vi "Read Menu Name.vi"(8 "error in":errorcluster, 11 "Standard Engine Editor Node in":refnum<class "Standard Engine Editor Node.lvclass">) -> (0 "error out":errorcluster, 2 "Name":string, 3 "Standard Engine Editor Node out":refnum<class "Standard Engine Editor Node.lvclass">)   [LabVIEW 2013, in "Standard Engine Editor Node.lvclass"]
uses:
  Standard Engine Editor Node.lvclass
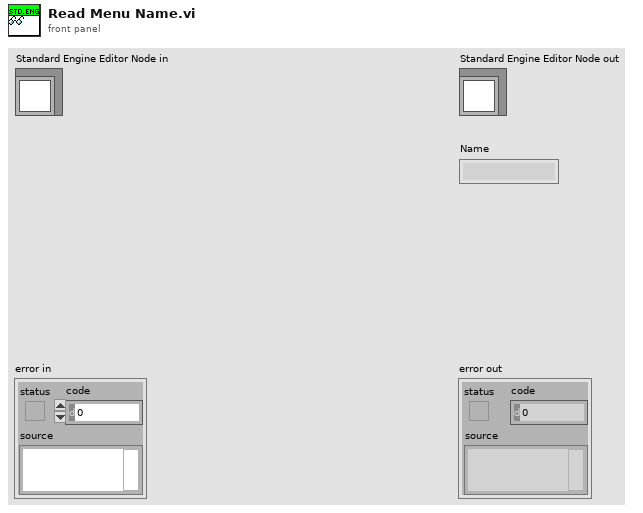
[diagram p1: front panel]
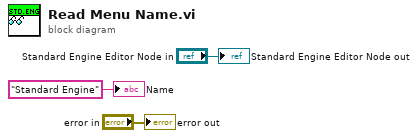
[diagram p0: block diagram]
diagram:
  "error out" <- "error in"
  "Standard Engine Editor Node out" <- "Standard Engine Editor Node in"
  "Name" <- "Standard Engine" ("Name")
